vi "Teaching View Facade.vi"(0 "Data In":T4, 2 "Display State In":T2={"Numeric"=0.0, "Fill Plots"=FALSE, "Cursor Redraw"=TRUE, "XYGraph Refnum"=refnum}, 3 "Container State":T3) -> (6 "Data Out":T4, 7 "Display State Out":T2={"Numeric"=0.0, "Fill Plots"=FALSE, "Cursor Redraw"=TRUE, "XYGraph Refnum"=refnum}, 8 "Action":T1)   [LabVIEW 2015, in "Teaching View.lvlib" / "Teaching View XControl.xctl"]
uses:
  Teaching View XControl.xctl
  Teaching View Data.ctl
  <vilib>/_xctls/Container State.ctl
  Teaching View State.ctl
  <vilib>/_xctls/Action.ctl
  <vilib>/_xctls/XControlSupport.lvlib
panel:
  out "XY Graph":cluster{"Data 2":dbl, u8}[](graph)
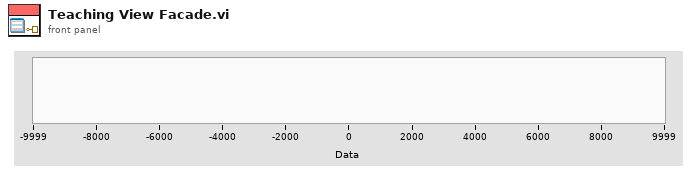
[diagram p1: front panel]
types:
  T1 = typedef "XControlSupport.lvlib/Action.ctl" = cluster{"Data Changed?":bool, "State Changed?":bool, "Action Name":string}
  T2 = typedef "Teaching View.lvlib/Teaching View XControl.xctl/Teaching View State.ctl" = cluster{"Numeric":dbl, "Fill Plots":bool, "Cursor Redraw":bool, "XYGraph Refnum":refnum<vi>}
  T3 = typedef "XControlSupport.lvlib/Container State.ctl" = cluster{"Indicator?":bool, "Run Mode?":bool, " Refnum":refnum<vi>}
  T4 = typedef "Teaching View.lvlib/Teaching View XControl.xctl/Teaching View Data.ctl" = cluster{"Upper Limit":dbl, "Lower Limit":dbl, "Measure":dbl[]}
  T5 = enum16{"Move", "left cursor", "right cursor", "none"}
  T6 = cluster{"Cursor Span":dbl, "Icon":u16, "Mouse Down":bool, "Owning VI":refnum<vi>, "Mouse area":enum16{"Move", "left cursor", "right cursor", "none"}, "Dragging":bool, "Drag Offset":dbl, "Original Cursor Pos":cluster{"Left":dbl, "Right":dbl, "Span":dbl}, "Cursor Redraw":bool}
  T7 = typedef "LVPoint32TypeDef.ctl" = cluster{"Horizontal":i32, "Vertical":i32}
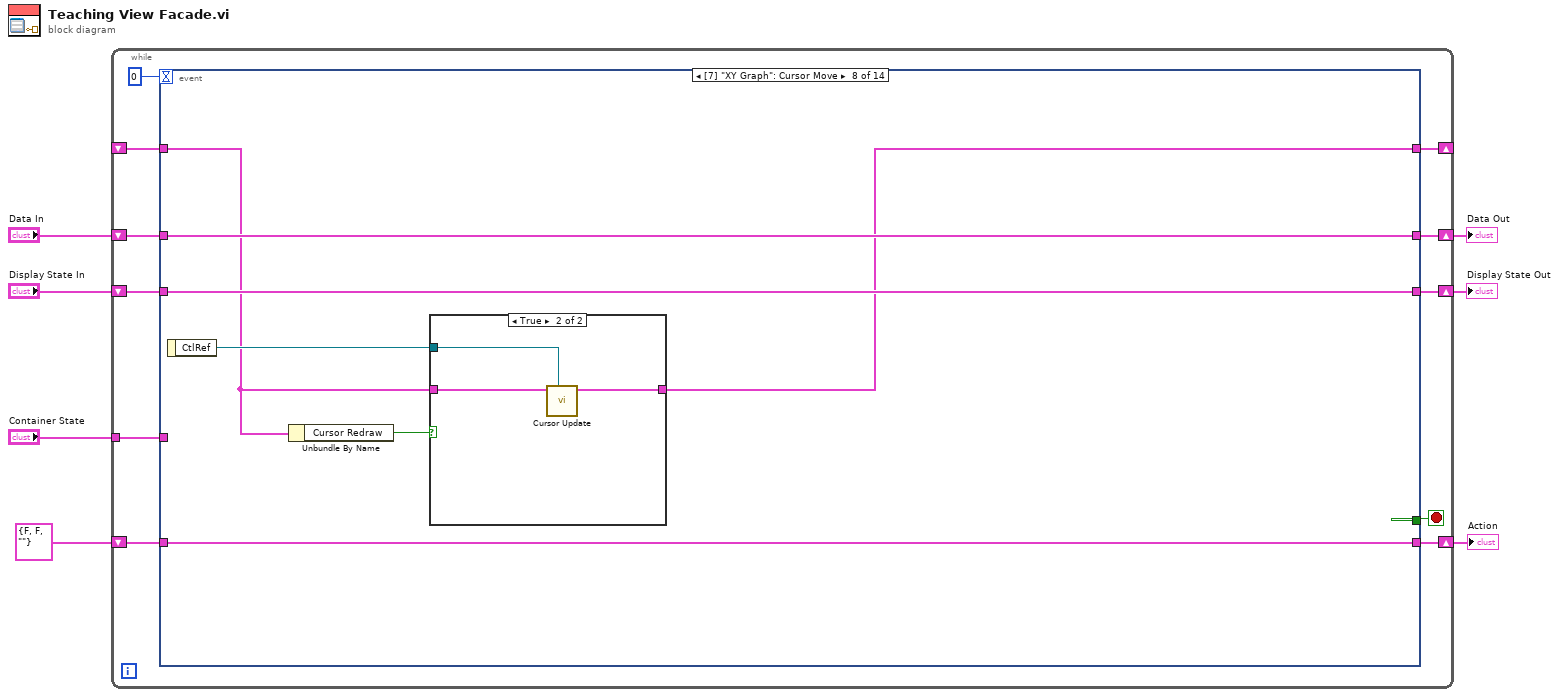
[diagram p0: block diagram]
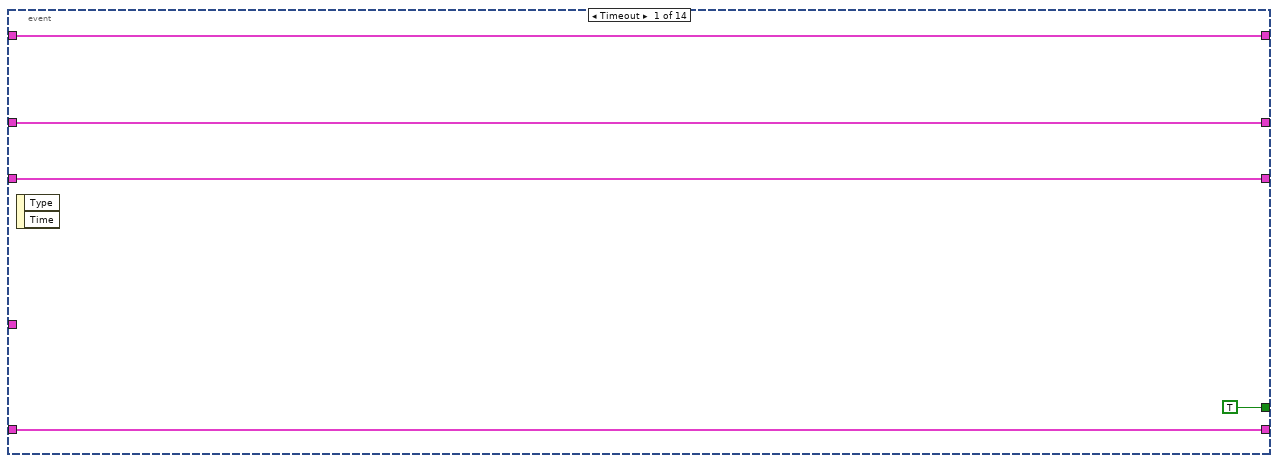
[diagram p2: hidden frame]
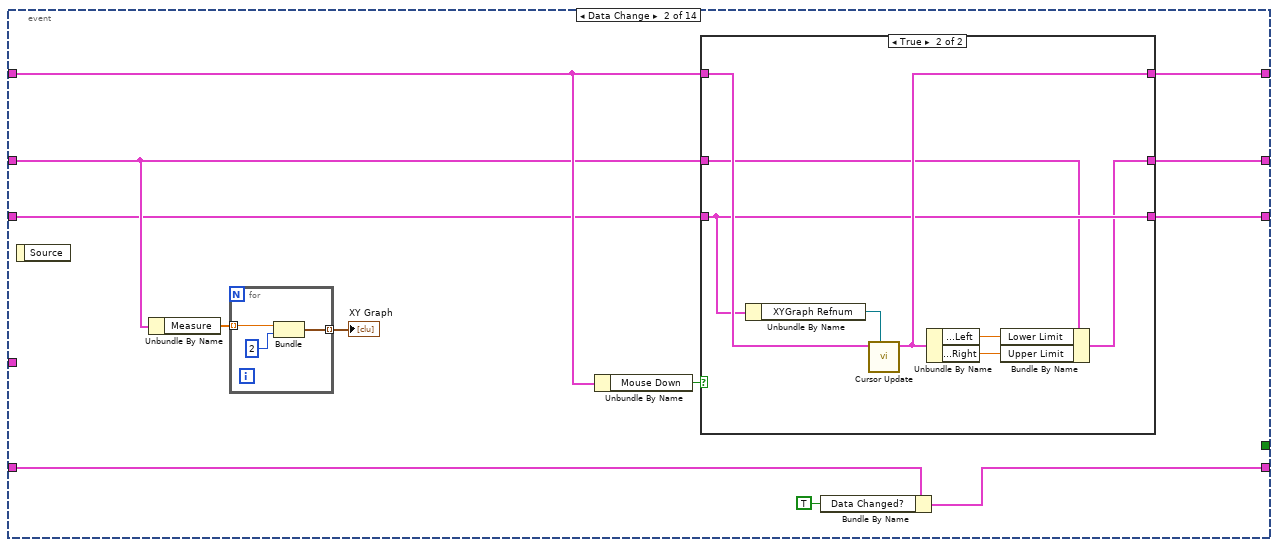
[diagram p3: hidden frame]
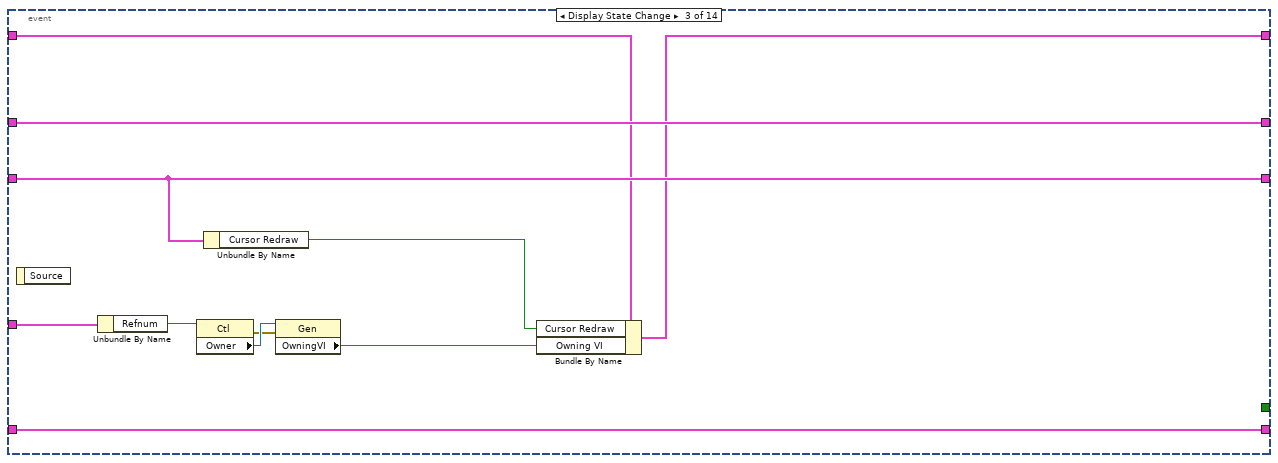
[diagram p5: hidden frame]
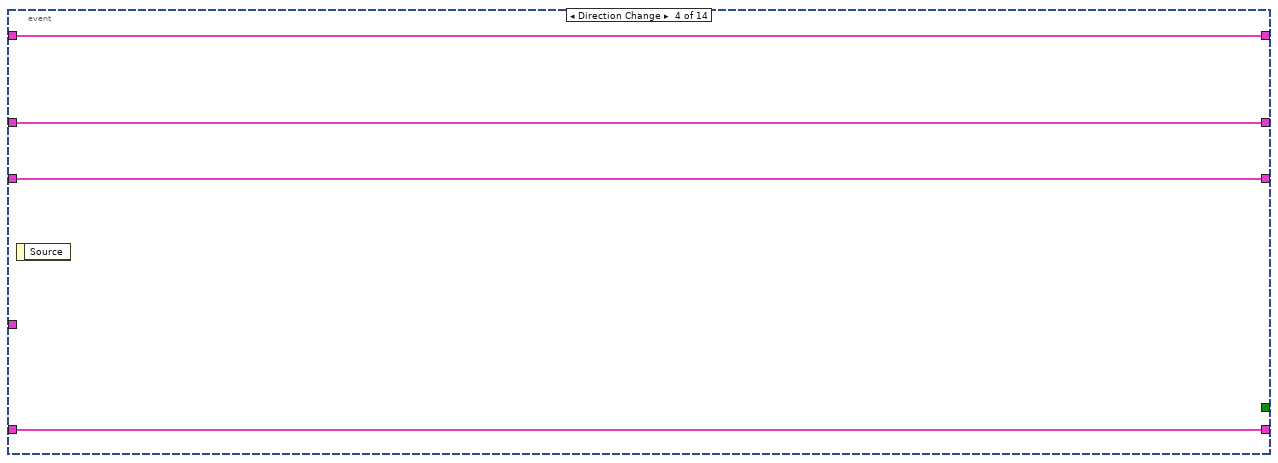
[diagram p6: hidden frame]
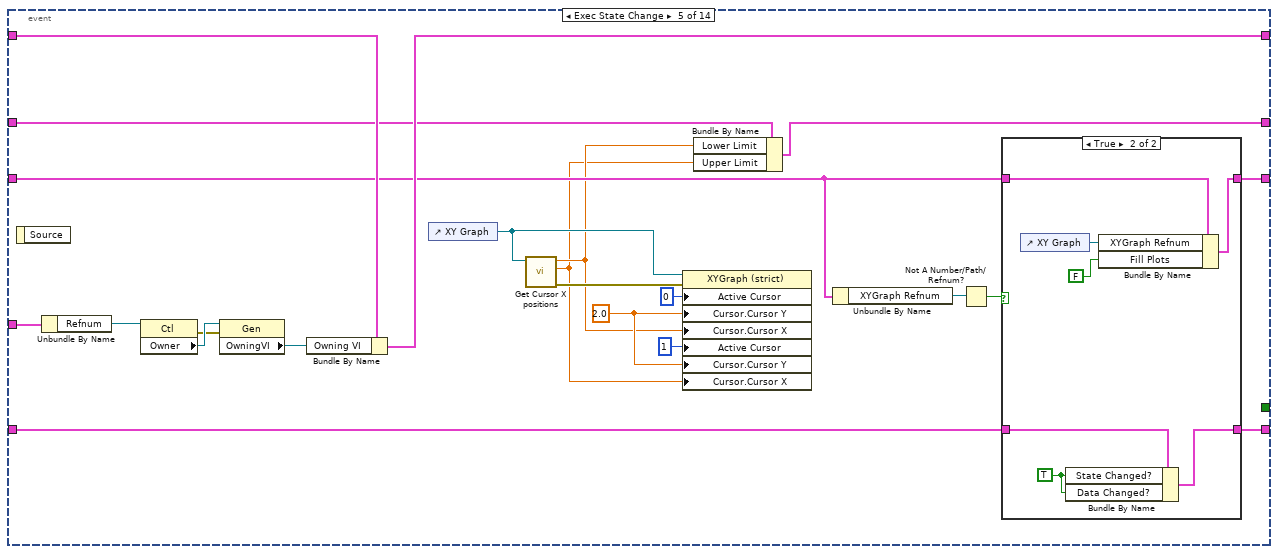
[diagram p7: hidden frame]
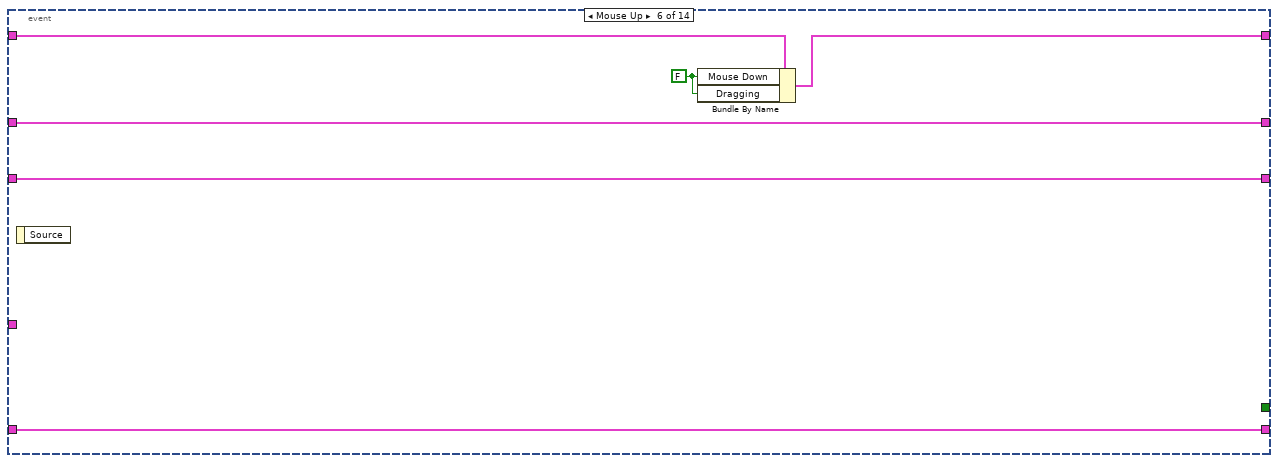
[diagram p9: hidden frame]
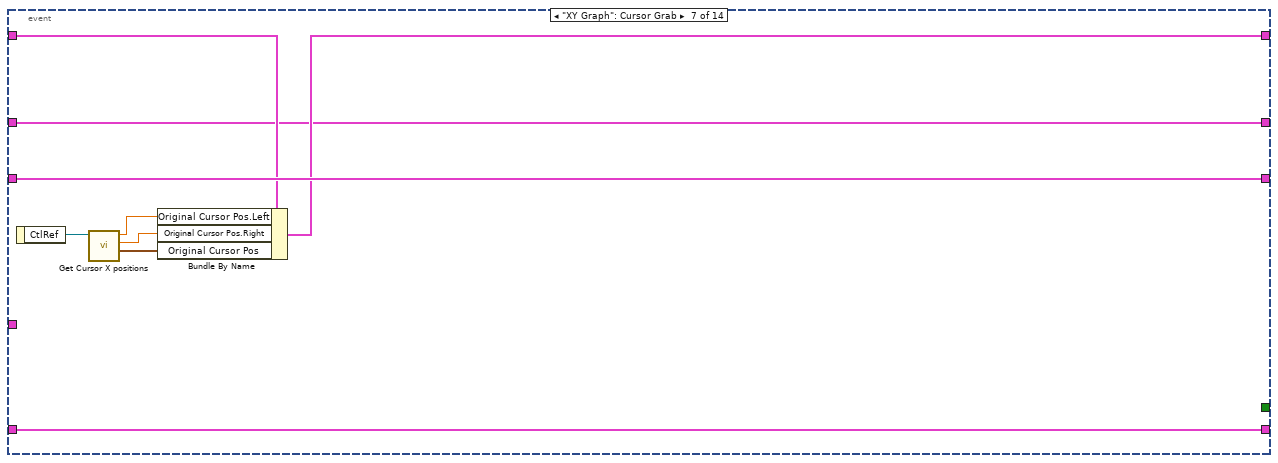
[diagram p10: hidden frame]
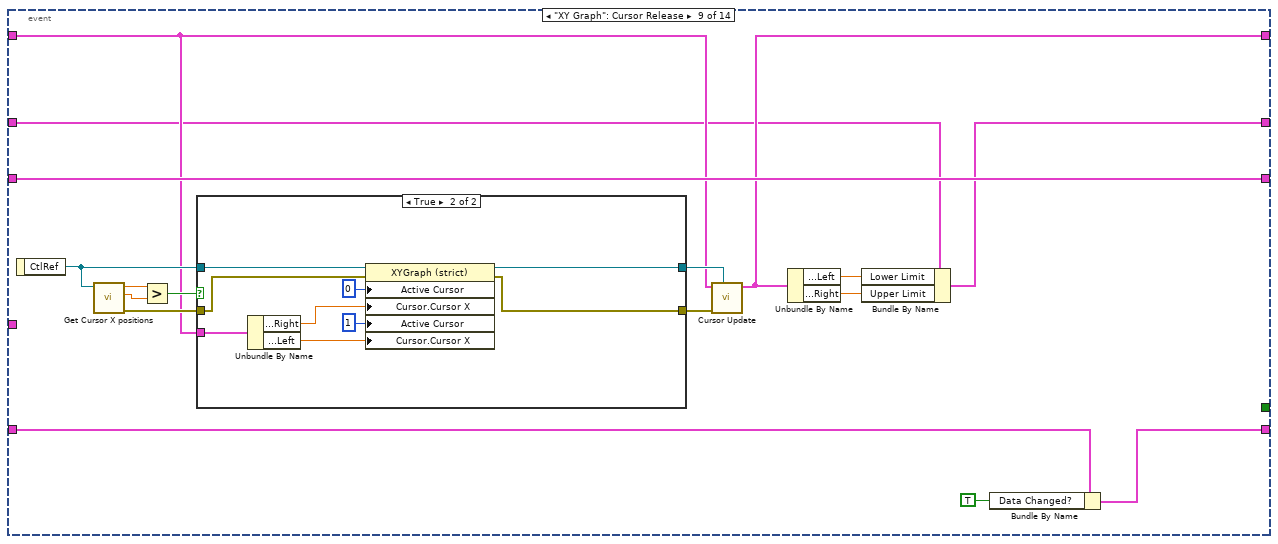
[diagram p12: hidden frame]
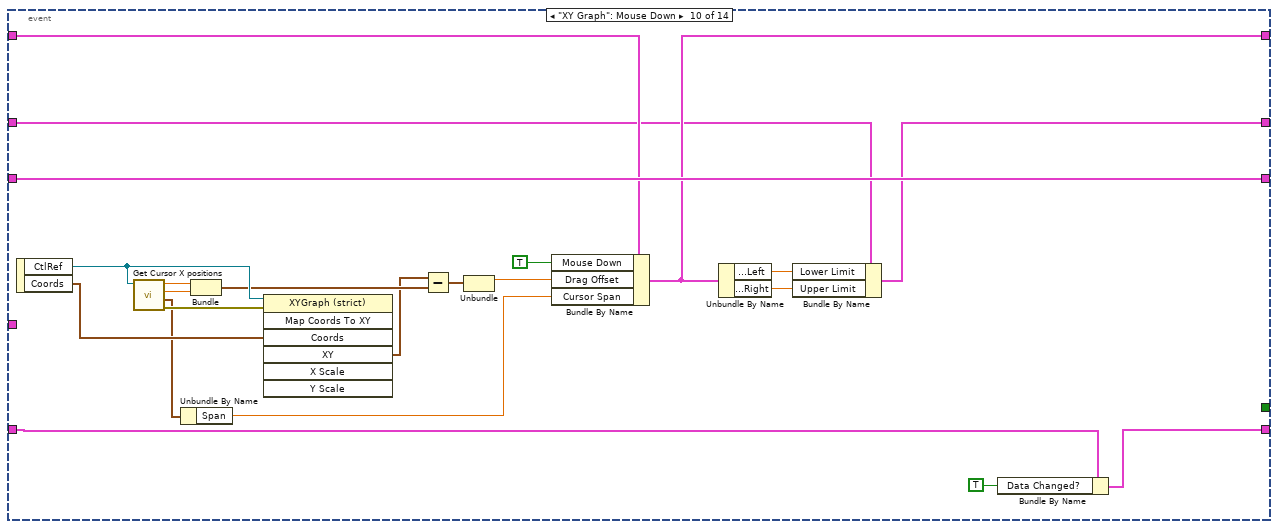
[diagram p14: hidden frame]
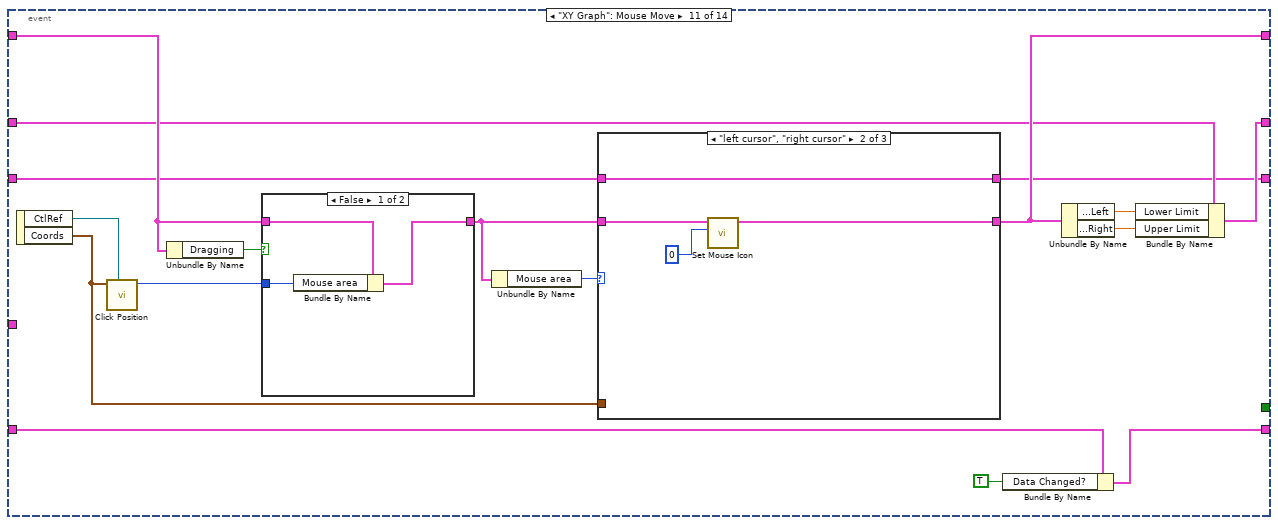
[diagram p15: hidden frame]
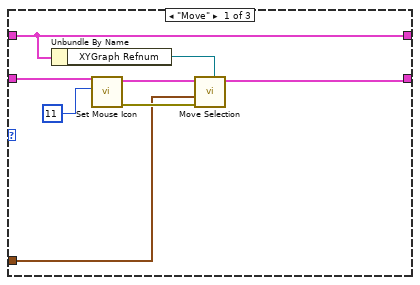
[diagram p16: hidden frame]
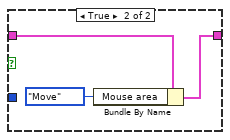
[diagram p18: hidden frame]
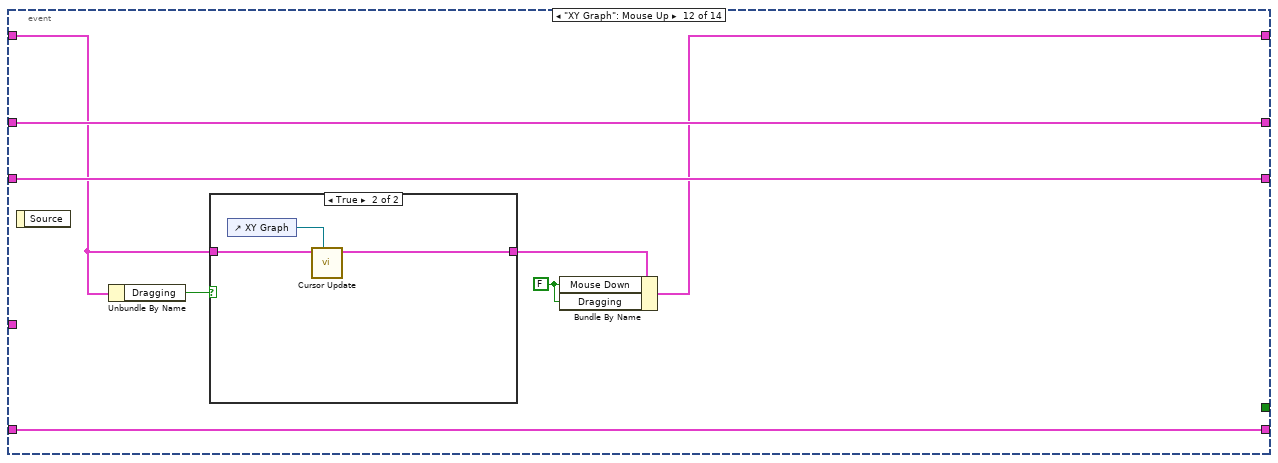
[diagram p19: hidden frame]
diagram:
  n1 = while {
    shift-right: [w17] -> w4
    shift-left: "Display State In" -> [w18]
    tunnel: "Container State" -> [w14]
    shift-right: [w12] -> w7
    shift-left: "Data In" -> [w13]
    shift-right: [w10] -> w2
    shift-left: T1 {"Data Changed?"=FALSE, "State Changed?"=FALSE, "Action Name"=""} ("Action") -> [w11]
    shift-right: [w9] -> _
    shift-left: _ -> [w8]
    stop <- w16 stop-if-true
    n2 = event shown="[7] \"XY Graph\": Cursor Move" {
      selector: _ -> [_ _ _ _ _ _ _ _ _ _ _ _ _ _]
      dyn-events: _ -> [_ _ _ _ _ _ _ _ _ _ _ _ _ _]
      timeout: 0 -> [_ _ _ _ _ _ _ _ _ _ _ _ _ _]
      tunnel: w18 -> [w21 w25 w53 w62 w73 w101 w110 w117 w138 w171 w173 w216 w226 w235]
      tunnel: [w21 w24 w53 w62 w72 w101 w110 w117 w138 w171 w172 w216 w226 w235] -> w17
      tunnel: [TRUE _ _ _ _ _ _ _ _ _ _ _ _ _] -> w16
      tunnel: w14 -> [_ _ w54 _ w83 _ _ _ _ _ _ _ _ _]
      tunnel: w13 -> [w20 w27 w60 w64 w68 w100 w102 w116 w128 w154 w178 w215 w225 w227]
      tunnel: [w20 w26 w60 w64 w65 w100 w102 w116 w125 w153 w177 w215 w225 w227] -> w12
      tunnel: [w22 w31 w59 w63 w71 w99 w109 w115 w122 w150 w174 w214 w224 w234] -> w10
      tunnel: w11 -> [w22 w33 w59 w63 w74 w99 w109 w115 w123 w151 w175 w214 w224 w234]
      tunnel: [w19 w28 w51 w61 w80 w96 w105 w111 w129 w155 w179 w209 w221 w228] -> w9
      tunnel: w8 -> [w19 w30 w52 w61 w82 w97 w107 w112 w131 w158 w187 w212 w223 w228]
      event Timeout {
        n3 = event-data() -> ()  [unwired: 1 in, 2 out]
      }
      event Data Change {
        n4 = event-data() -> ()  [unwired: 1 in, 1 out]
        n5 = Unbundle By Name(w27) -> ("Measure"=w35:dbl[])
        n6 = for {
          tunnel: w35 -> [w49] mode=indexing
          tunnel: [w47] -> w34 mode=indexing
          n7 = Bundle("Data 2"=w49, u8 2) -> (w47:cluster{"Data 2":dbl, u8})  [unwired: 1 in]
        }
        "XY Graph" <- w34
        n8 = Unbundle By Name(w30) -> ("Mouse Down"=w29:bool)
        n9 = case shown="True" w29 {
          tunnel: w30 -> [w38 w44]
          tunnel: [w38 w43] -> w28
          tunnel: w27 -> [w37 w40]
          tunnel: [w37 w39] -> w26
          tunnel: w25 -> [w36 w41]
          tunnel: [w36 w41] -> w24
          frame False {
          }
          frame True {
            n10 = Unbundle By Name(w41) -> ("XYGraph Refnum"=w42:refnum<vi>)
            n11 = call "Cursor Update.vi"("XY Graph Ref"=w42, "Xinformation In"=w44) -> ("Xinformation Out"=w43:T6)  [unwired: 8 in, 1 out]
            n12 = Unbundle By Name(w43) -> ("Original Cursor Pos.Left"=w46:dbl, "Original Cursor Pos.Right"=w45:dbl)
            n13 = Bundle By Name(cluster=w40, "Lower Limit"=w46, "Upper Limit"=w45) -> (w39:T4)
          }
        }
        n14 = Bundle By Name(cluster=w33, "Data Changed?"=TRUE) -> (w31:T1)
      }
      event Display State Change {
        n15 = event-data() -> ()  [unwired: 1 in, 1 out]
        n16 = Unbundle By Name(w54) -> ("Refnum"=w57:refnum<vi>)
        n17 = property class="Ctl"(reference=w57) -> (error out=w56:errorcluster, "Owner"=w58:refnum<vi>)  [unwired: 1 in, 1 out]
        n18 = Unbundle By Name(w53) -> ("Cursor Redraw"=w50:bool)
        n19 = property class="Gen"(reference=w58, error in=w56) -> ("OwningVI"=w55:refnum<vi>)  [unwired: 2 out]
        n20 = Bundle By Name(cluster=w52, "Cursor Redraw"=w50, "Owning VI"=w55) -> (w51:T6)
      }
      event Direction Change {
        n21 = event-data() -> ()  [unwired: 1 in, 1 out]
      }
      event Exec State Change {
        w70 = 2.0
        n22 = event-data() -> ()  [unwired: 1 in, 1 out]
        n23 = Unbundle By Name(w83) -> ("Refnum"=w85:refnum<vi>)
        n24 = property class="Ctl"(reference=w85) -> (error out=w84:errorcluster, "Owner"=w86:refnum<vi>)  [unwired: 1 in, 1 out]
        n25 = property class="Gen"(reference=w86, error in=w84) -> ("OwningVI"=w81:refnum<vi>)  [unwired: 2 out]
        n26 = Bundle By Name(cluster=w82, "Owning VI"=w81) -> (w80:T6)
        n27 = control-ref of="XY Graph"() -> (w78:refnum<vi>)
        n28 = call "Get Cursor X positions.vi"("XY Graph Ref"=w78) -> ("error out"=w79:errorcluster, "Right"=w66:dbl, "Left"=w67:dbl)  [unwired: 7 in, 1 out]
        n29 = property class="XYGraph (strict)"(reference=w78, error in=w79, "Active Cursor"=u32 0, "Cursor.Cursor Y"=w70, "Cursor.Cursor X"=w67, "Active Cursor"=u32 1, "Cursor.Cursor Y"=w70, "Cursor.Cursor X"=w66) -> ()  [unwired: 2 out]
        n30 = Bundle By Name(cluster=w68, "Lower Limit"=w67, "Upper Limit"=w66) -> (w65:T4)
        n31 = Unbundle By Name(w73) -> ("XYGraph Refnum"=w76:refnum<vi>)
        n32 = Not A Number/Path/Refnum?(number/path/refnum=w76) -> (NaN/Path/Refnum?=w75:bool)
        n33 = case shown="True" w75 {
          tunnel: w74 -> [w87 w91]
          tunnel: w73 -> [w88 w95]
          tunnel: [w88 w92] -> w72
          tunnel: [w87 w90] -> w71
          frame False {
          }
          frame True {
            w89 = TRUE ("State Changed?")
            n34 = control-ref of="XY Graph"() -> (w94:refnum<vi>)
            n35 = Bundle By Name(cluster=w91, "State Changed?"=w89, "Data Changed?"=w89) -> (w90:T1)
            n36 = Bundle By Name(cluster=w95, "XYGraph Refnum"=w94, "Fill Plots"=FALSE) -> (w92:T2)
          }
        }
      }
      event Mouse Up {
        w98 = FALSE ("Mouse Down")
        n37 = event-data() -> ()  [unwired: 1 in, 1 out]
        n38 = Bundle By Name(cluster=w97, "Mouse Down"=w98, "Dragging"=w98) -> (w96:T6)
      }
      event "XY Graph": Cursor Grab {
        n39 = event-data() -> ("CtlRef"=w108:refnum<vi>)  [unwired: 1 in]
        n40 = call "Get Cursor X positions.vi"("XY Graph Ref"=w108) -> ("Cursors"=w106:cluster{"Left":dbl, "Right":dbl, "Span":dbl}, "Right"=w103:dbl, "Left"=w104:dbl)  [unwired: 7 in, 1 out]
        n41 = Bundle By Name(cluster=w107, "Original Cursor Pos.Left"=w104, "Original Cursor Pos.Right"=w103, "Original Cursor Pos"=w106) -> (w105:T6)
      }
      event "XY Graph": Cursor Move {
        n42 = event-data() -> ("CtlRef"=w113:refnum<vi>)  [unwired: 1 in]
        n43 = Unbundle By Name(w112) -> ("Cursor Redraw"=w114:bool)
        n44 = case shown="True" w114 {
          tunnel: w113 -> [_ w121]
          tunnel: w112 -> [w118 w120]
          tunnel: [w118 w119] -> w111
          frame False {
          }
          frame True {
            n45 = call "Cursor Update.vi"("XY Graph Ref"=w121, "Xinformation In"=w120) -> ("Xinformation Out"=w119:T6)  [unwired: 8 in, 1 out]
          }
        }
      }
      event "XY Graph": Cursor Release {
        n46 = event-data() -> ("CtlRef"=w137:refnum<vi>)  [unwired: 1 in]
        n47 = call "Get Cursor X positions.vi"("XY Graph Ref"=w137) -> ("error out"=w133:errorcluster, "Right"=w135:dbl, "Left"=w136:dbl)  [unwired: 7 in, 1 out]
        n48 = Greater?(x=w136, y=w135) -> (0:w134:bool)
        n49 = case shown="True" w134 {
          tunnel: w137 -> [w140 w145]
          tunnel: w133 -> [w139 w144]
          tunnel: [w140 w143] -> w132
          tunnel: w131 -> [_ w142]
          tunnel: [w139 w141] -> w130
          frame False {
          }
          frame True {
            n50 = Unbundle By Name(w142) -> ("Original Cursor Pos.Right"=w148:dbl, "Original Cursor Pos.Left"=w149:dbl)
            n51 = property class="XYGraph (strict)"(reference=w145, error in=w144, "Active Cursor"=u32 0, "Cursor.Cursor X"=w148, "Active Cursor"=u32 1, "Cursor.Cursor X"=w149) -> (reference out=w143:refnum<vi>, error out=w141:errorcluster)
          }
        }
        n52 = call "Cursor Update.vi"("XY Graph Ref"=w132, "error in (no error)"=w130, "Xinformation In"=w131) -> ("Xinformation Out"=w129:T6)  [unwired: 7 in, 1 out]
        n53 = Unbundle By Name(w129) -> ("Original Cursor Pos.Left"=w127:dbl, "Original Cursor Pos.Right"=w126:dbl)
        n54 = Bundle By Name(cluster=w128, "Lower Limit"=w127, "Upper Limit"=w126) -> (w125:T4)
        n55 = Bundle By Name(cluster=w123, "Data Changed?"=TRUE ("State Changed?")) -> (w122:T1)
      }
      event "XY Graph": Mouse Down {
        n56 = event-data() -> ("CtlRef"=w169:refnum<vi>, "Coords"=w168:T7)  [unwired: 1 in]
        n57 = call "Get Cursor X positions.vi"("XY Graph Ref"=w169) -> ("error out"=w170:errorcluster, "Cursors"=w160:cluster{"Left":dbl, "Right":dbl, "Span":dbl}, "Right"=w166:dbl, "Left"=w167:dbl)  [unwired: 7 in]
        n58 = Unbundle By Name(w160) -> ("Span"=w159:dbl)
        n59 = Bundle("Left"=w167, "Right"=w166) -> (w165:cluster{"Left":dbl, "Right":dbl})  [unwired: 1 in]
        n60 = invoke on="Invoke Node" class="XYGraph (strict)" method="Map Coords To XY"(reference=w169, error in=w170, "Coords"=w168) -> ("XY"=w164:cluster{"X":dbl, "Y":dbl})  [unwired: 4 in, 6 out]
        n61 = Subtract(x=w164, y=w165) -> (x-y=w161:cluster{dbl, dbl})
        n62 = Unbundle(w161) -> (w163:dbl)  [unwired: 1 out]
        n63 = Bundle By Name(cluster=w158, "Mouse Down"=TRUE, "Drag Offset"=w163, "Cursor Span"=w159) -> (w155:T6)
        n64 = Unbundle By Name(w155) -> ("Original Cursor Pos.Left"=w157:dbl, "Original Cursor Pos.Right"=w156:dbl)
        n65 = Bundle By Name(cluster=w154, "Lower Limit"=w157, "Upper Limit"=w156) -> (w153:T4)
        n66 = Bundle By Name(cluster=w151, "Data Changed?"=TRUE ("State Changed?")) -> (w150:T1)
      }
      event "XY Graph": Mouse Move {
        n67 = event-data() -> ("CtlRef"=w182:refnum<vi>, "Coords"=w184:T7)  [unwired: 1 in]
        n68 = call "Click Position.vi"("XY Graph Ref"=w182, "Click Coords"=w184) -> ("Operation"=w183:T5)  [unwired: 8 in, 1 out]
        n69 = Unbundle By Name(w187) -> ("Dragging"=w188:bool)
        n70 = case shown="False" w188 {
          tunnel: w187 -> [w205 w208]
          tunnel: w183 -> [w204 _]
          tunnel: [w203 w206] -> w185
          frame False {
            n71 = Bundle By Name(cluster=w205, "Mouse area"=w204) -> (w203:T6)
          }
          frame True {
            n72 = Bundle By Name(cluster=w208, "Mouse area"=T5."Move") -> (w206:T6)
          }
        }
        n73 = Unbundle By Name(w185) -> ("Mouse area"=w186:T5)
        n74 = case shown="\"left cursor\", \"right cursor\"" w186 {
          tunnel: w185 -> [w195 w200 w202]
          tunnel: [w192 w198 w202] -> w179
          tunnel: w184 -> [w191 _ _]
          tunnel: w173 -> [w190 w197 w201]
          tunnel: [w190 w197 w201] -> w172
          frame "Move" {
            n75 = Unbundle By Name(w190) -> ("XYGraph Refnum"=w189:refnum<vi>)
            n76 = call "Set Mouse Icon.vi"("icon"=u16 11, "Xinformation In"=w195) -> ("error out"=w194:errorcluster, "Xinformation Out"=w193:T6)  [unwired: 8 in]
            n77 = call "Move Selection.vi"("XY Graph Ref"=w189, "error in (no error)"=w194, "Coords"=w191, "Xinformation In"=w193) -> ("Xinformation Out"=w192:T6)  [unwired: 6 in, 1 out]
          }
          frame "left cursor", "right cursor" {
            n78 = call "Set Mouse Icon.vi"("icon"=u16 0, "Xinformation In"=w200) -> ("Xinformation Out"=w198:T6)  [unwired: 8 in, 1 out]
          }
          frame "none", Default {
          }
        }
        n79 = Bundle By Name(cluster=w175, "Data Changed?"=TRUE ("State Changed?")) -> (w174:T1)
        n80 = Unbundle By Name(w179) -> ("Original Cursor Pos.Left"=w181:dbl, "Original Cursor Pos.Right"=w180:dbl)
        n81 = Bundle By Name(cluster=w178, "Lower Limit"=w181, "Upper Limit"=w180) -> (w177:T4)
      }
      event "XY Graph": Mouse Up {
        w211 = FALSE
        n82 = event-data() -> ()  [unwired: 1 in, 1 out]
        n83 = Unbundle By Name(w212) -> ("Dragging"=w213:bool)
        n84 = case shown="True" w213 {
          tunnel: w212 -> [w217 w220]
          tunnel: [w217 w218] -> w210
          frame False {
          }
          frame True {
            n85 = control-ref of="XY Graph"() -> (w219:refnum<vi>)
            n86 = call "Cursor Update.vi"("XY Graph Ref"=w219, "Xinformation In"=w220) -> ("Xinformation Out"=w218:T6)  [unwired: 8 in, 1 out]
          }
        }
        n87 = Bundle By Name(cluster=w210, "Mouse Down"=w211, "Dragging"=w211) -> (w209:T6)
      }
      event "XY Graph": Mouse Leave {
        n88 = event-data() -> ()  [unwired: 1 in, 1 out]
        n89 = call "Set Mouse Icon.vi"("icon"=u16 0, "Xinformation In"=w223) -> ("Xinformation Out"=w221:T6)  [unwired: 8 in, 1 out]
      }
      event "XY Graph": Scale Range Change {
        n90 = event-data() -> ("CtlRef"=w233:refnum<vi>)  [unwired: 1 in]
        n91 = Unbundle By Name(w228) -> ("Original Cursor Pos.Left"=w230:dbl, "Original Cursor Pos.Right"=w229:dbl)
        n92 = property class="XYGraph (strict)"(reference=w233, "Active Cursor"=u32 0, "Cursor.Cursor X"=w230, "Active Cursor"=u32 1, "Cursor.Cursor X"=w229) -> ()  [unwired: 1 in, 2 out]
      }
    }
  }
  "Display State Out" <- w4
  "Data Out" <- w7
  "Action" <- w2
